vi "img_write_file_header.vi"(4 "Y count":u32=1, 6 "X count":u32=1, 7 "Frame Count":u32, 8 "error in":errorcluster, 9 "sector size (512)":u32=512, 10 "Image In":T1, 11 "hFile":i64) -> (0 "error out":errorcluster, 1 "lpNumberOfBytesWritten":u32, 2 "Image Out":T1, 3 "hFile out":i64)   [LabVIEW 2016]
doc: "This VI writes header information to file describing the image properties. The header is one disk sector in size (often 512 bytes). Each field is 4 bytes:\n\n1) X resolution\n2) Y resolution\n3) Image type\n4) Image border size\n5) Linewidth (pixels)\n6) Bytes per pixel\n7) Number of images in X direction\n8) Number of images in Y direction"
uses:
  <vilib>/vision/Image Controls.llb/IMAQ Image.ctl
  kernel32.dll
panel:
  out "Y Resolution":i32
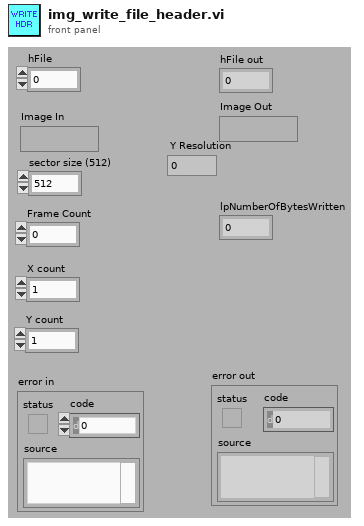
[diagram p1: front panel]
types:
  T1 = typedef "IMAQ Image.ctl" = refnum<image>
  T2 = enum32{"Map Pixel Pointer", "Unmap Pixel Pointer", "Get Pixels Infos"}
  T3 = typedef "Image Type" = u32
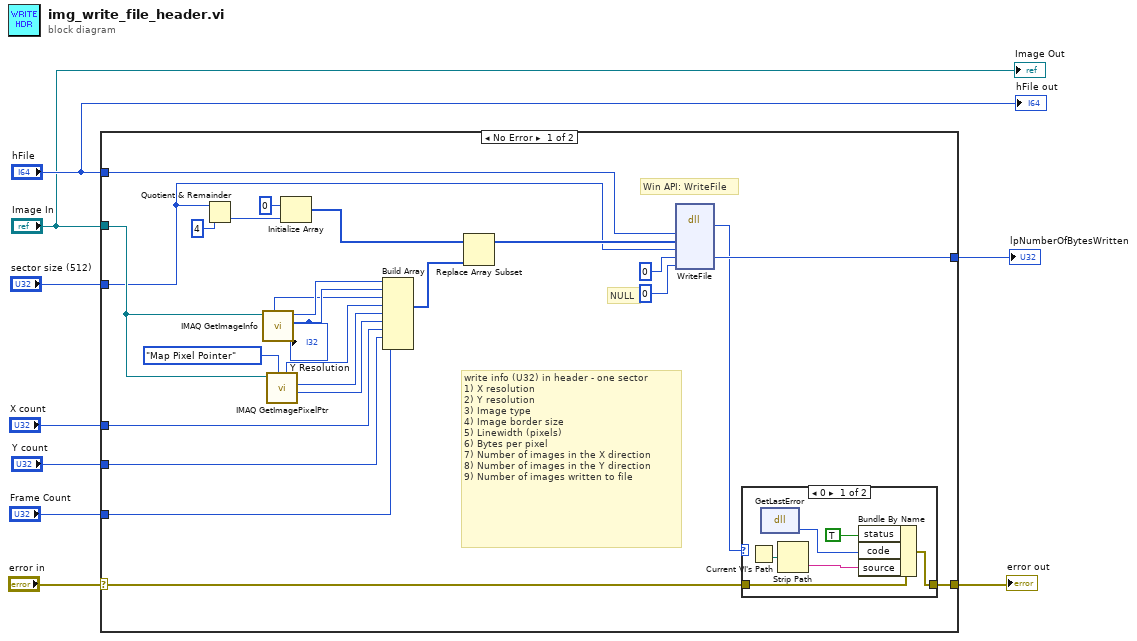
[diagram p0: block diagram]
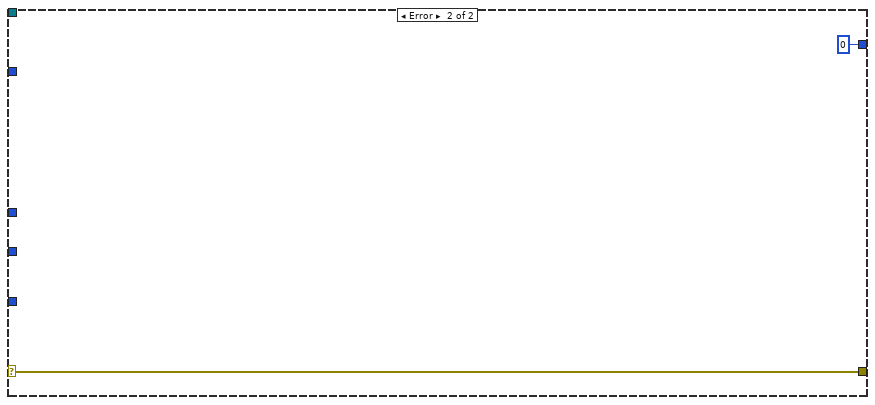
[diagram p3: hidden frame]
diagram:
  n1 = case shown="No Error" "error in" {
    selector: "error in" -> [w26 w42]
    tunnel: "hFile" -> [w32 _]
    tunnel: "Image In" -> [w29 _]
    tunnel: [w30 u32 0 ("lpNumberOfBytesWritten")] -> w7
    tunnel: [w28 w42] -> w6
    tunnel: "sector size (512)" -> [w13 _]
    tunnel: "X count" -> [w12 _]
    tunnel: "Y count" -> [w11 _]
    tunnel: "Frame Count" -> [w10 _]
    frame No Error {
      # "write info (U32) in header - one sector\n1) X resolution\n2) Y resolution\n3) Image type\n4) Image border size\n5) Linewidth (pixels)\n6) Bytes per pixel\n7) Number of images in the X direction\n8) Number of images in the Y direction\n9) Number of images written to file"
      # "Win API: WriteFile"
      # "NULL"
      n2 = Quotient & Remainder(x=w13, y=u32 4 ("element")) -> (floor(x/y)=w23:u32)  [unwired: 1 out]
      n3 = call "IMAQ GetImageInfo"("Image"=w29) -> ("Y Resolution"=w21:i32, "X Resolution"=w22:i32, "Image Type"=w20:T3)  [unwired: 1 in, 7 out]
      "Y Resolution" <- w21
      n4 = call "IMAQ GetImagePixelPtr"("Function"=T2."Map Pixel Pointer", "Image"=w29) -> ("Pixel Size (Bytes)"=w17:i32, "LineWidth(Pixels)"=w18:i32, "Image Border Size"=w19:i32)  [unwired: 4 in, 3 out]
      n5 = Initialize Array(u32 0 ("element"), w23) -> (w15:u32[])
      n6 = Build Array(w22, w21, w20, w19, w18, w17, w12, w11, w10) -> (w16:T3[])
      n7 = Replace Array Subset(array=w15, new element=w16) -> (w14:u32[])  [unwired: 1 in]
      n8 = dll-call lib="kernel32.dll" fn="WriteFile"("hFile"=w32, "lpBuffer"=w14, "nNumberOfBytesToWrite"=w13, "lpNumberOfBytesWritten"=u32 0, "lpOverlapped"=u32 0) -> ("error"=w25:i32, "lpNumberOfBytesWritten"=w30:u32)  [unwired: 7 in, 2 out]
      n9 = case shown="0" w25 {
        tunnel: w26 -> [w40 w41]
        tunnel: [w39 w41] -> w28
        frame 0 {
          n10 = Current VI's Path() -> (path=w37:path)
          n11 = dll-call lib="kernel32.dll" fn="GetLastError"() -> ("error"=w35:u32)  [unwired: 3 in, 2 out]
          n12 = Strip Path(path=w37) -> (name=w36:string)  [unwired: 1 out]
          n13 = Bundle By Name(cluster=w40, "status"=TRUE, "code"=w35, "source"=w36) -> (w39:errorcluster)
        }
        frame 1, Default {
        }
      }
    }
    frame Error {
    }
  }
  "lpNumberOfBytesWritten" <- w7
  "error out" <- w6
  "Image Out" <- "Image In"
  "hFile out" <- "hFile"
